vi "Command Handler (8 Bits).vi"(9 "operation":u32 format="%.0x", 11 "device connection map in":T2={"RS"="RS", "R/W"="RW", "E1"="E1", "E2"="E1", "DB0"="DB0", "DB1"="DB1", "DB2"="DB2", "DB3"="DB3", "DB4"="DB4", "DB5"="DB5", "DB6"="DB6", "DB7"="DB7"}) -> (3 "result":T1)   [LabVIEW 2017, in "HD44780 FPGA.lvlib"]
doc: "Receives and parses commands from the Host VIs or FPGA VIs."
uses:
  HD44780 FPGA.lvlib
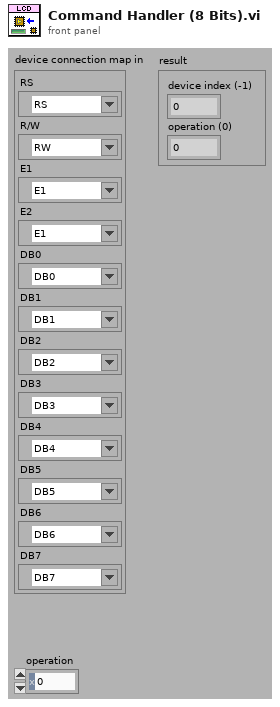
[diagram p1: front panel]
types:
  T1 = cluster{"device index (-1)":i8, "operation (0)":u32}
  T2 = cluster{"RS":refnum<k21>, "R/W":refnum<k21>, "E1":refnum<k21>, "E2":refnum<k21>, "DB0":refnum<k21>, "DB1":refnum<k21>, "DB2":refnum<k21>, "DB3":refnum<k21>, "DB4":refnum<k21>, "DB5":refnum<k21>, "DB6":refnum<k21>, "DB7":refnum<k21>}
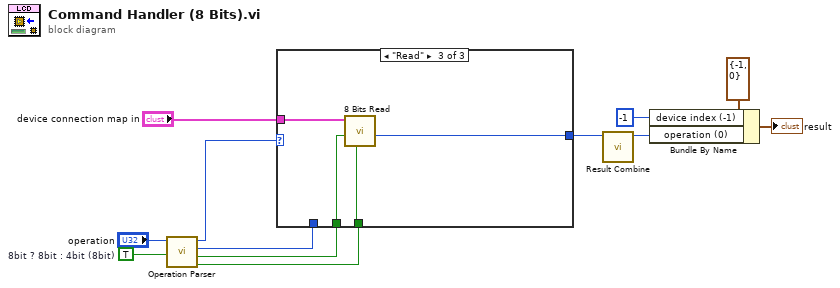
[diagram p0: block diagram]
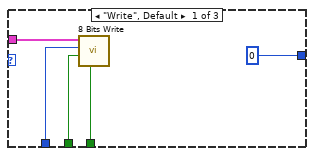
[diagram p2: hidden frame]
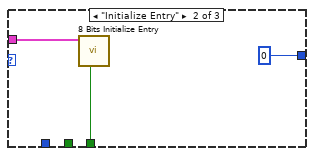
[diagram p3: hidden frame]
diagram:
  w5 = TRUE  # 8bit ? 8bit : 4bit (8bit)
  n1 = call "Operation Parser.vi"("8bit ? 8bit : 4bit (8bit)"=w5, "operation"="operation") -> ("E1? E1: E2 (E1)"=w6:bool, "RS"=w7:bool, "cmd/data"=w8:u8, "command type"=w11:enum8{"Write", "Read", "Initialize Entry"})  [unwired: 6 in]
  n2 = case shown="\"Read\"" w11 {
    tunnel: "device connection map in" -> [w13 w19 w24]
    tunnel: [u8 0 ("value") u8 0 ("value") w23] -> w9
    tunnel: w8 -> [w17 _ _]
    tunnel: w7 -> [w16 _ w22]
    tunnel: w6 -> [w15 w18 w21]
    frame "Write", Default {
      n3 = call "8 Bits Write.vi"("E?E1:E2 (E1)"=w15, "RS"=w16, "LCD data/cmd"=w17, "device connection map"=w13) -> ()  [unwired: 8 in]
    }
    frame "Initialize Entry" {
      n4 = call "8 Bits Initialize Entry.vi"("E?E1:E2 (E1)"=w18, "device connection map"=w19) -> ()  [unwired: 10 in]
    }
    frame "Read" {
      n5 = call "8 Bits Read.vi"("E?E1:E2 (E1)"=w21, "RS"=w22, "device connection map"=w24) -> ("value"=w23:u8)  [unwired: 8 in]
    }
  }
  n6 = call "Result Combine.vi"("content"=w9) -> ("result"=w3:u32)  [unwired: 10 in]
  n7 = Bundle By Name(cluster=T1 {"device index (-1)"=-1, "operation (0)"=0} ("LCD Command"), "device index (-1)"=i8 -1 ("device index"), "operation (0)"=w3) -> (→"result":T1)
